vi "Set Write Timeout.vi"(8 "error in (no error)":errorcluster, 10 "write operation timeout":i32=5000, 11 "Modbus master in":refnum<class "Modbus Master.lvclass">) -> (0 "error out":errorcluster, 3 "Modbus master out":refnum<class "Modbus Master.lvclass">)   [LabVIEW 2017, in "Modbus Master.lvclass"]
doc: "<B>Write Timeout</B> specifies the write operation timeout. You can use a Modbus master instance to perform write operations on a Modbus slave with the specified timeout."
uses:
  <vilib>/Modbus/master/Modbus Master.lvclass
  C:/builds/penguin/iak/lvdsc/trunk/17.0/lv/vi.lib/Modbus/subvis/Modbus API/Modbus API.lvclass
  <vilib>/Modbus/subvis/Modbus API/Modbus API.lvclass/Modbus API.ctl
  <vilib>/Modbus/subvis/Transmission Data Unit (ADU)/Transmission Data Unit/Transmission Data Unit.lvclass/Transmission Data Unit.ctl
  <vilib>/Modbus/subvis/Transmission Data Unit (ADU)/Transmission Data Unit/Transmission Data Unit.lvclass
  <vilib>/Modbus/subvis/Modbus API/Modbus API.lvclass
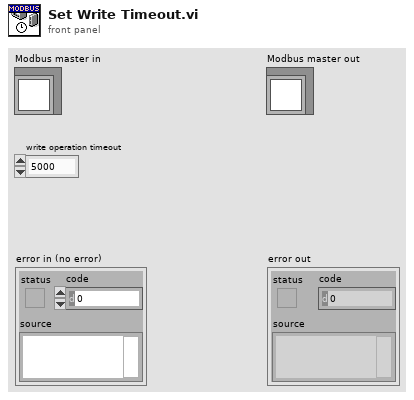
[diagram p1: front panel]
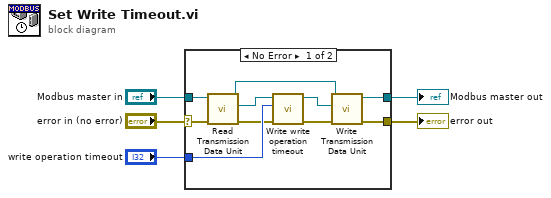
[diagram p0: block diagram]
diagram:
  n1 = case shown="No Error" "error in (no error)" {
    selector: "error in (no error)" -> [w6 w17]
    tunnel: "write operation timeout" -> [w12 _]
    tunnel: "Modbus master in" -> [w11 w16]
    tunnel: [w10 w16] -> w3
    tunnel: [w9 w17] -> w2
    frame No Error {
      n2 = call <vilib>:"Read Transmission Data Unit.vi"("error in (no error)"=w6, "Modbus instance in"=w11) -> ("error out"=w7:errorcluster, "transmission data unit"=w13:refnum<class "Transmission Data Unit.lvclass">, "Modbus instance out"=w15:refnum<class "Modbus Master.lvclass">)  [unwired: 7 in]
      n3 = call <vilib>:"Write write operation timeout.vi"("error in (no error)"=w7, "write operation timeout"=w12, "transmission data unit in"=w13) -> ("error out"=w8:errorcluster, "transmission data unit out"=w14:refnum<class "Transmission Data Unit.lvclass">)  [unwired: 7 in]
      n4 = call <vilib>:"Write Transmission Data Unit.vi"("error in (no error)"=w8, "transmission data unit"=w14, "Modbus instance in"=w15) -> ("error out"=w9:errorcluster, "Modbus instance out"=w10:refnum<class "Modbus Master.lvclass">)  [unwired: 7 in]
    }
    frame Error {
    }
  }
  "error out" <- w2
  "Modbus master out" <- w3
